vi "HeaderAction.vi"(0 "InstrClass":refnum<class "CoboltMLD.lvclass"> caption="DNL_LabVIEW Object in", 11 "error in (no error)":errorcluster caption="entrée d'erreur (pas d'erreur)") -> (4 "InstrClassOut":refnum<class "CoboltMLD.lvclass"> caption="DNL_LabVIEW Object out", 6 "DataNames":string[](array[string]), 8 "Instr Name":string, 10 "HeaderString":string, 13 "ArrDisplayNames":string[](array[string]), 14 "DisplayNames":string[](array[string]), 15 "error out":errorcluster caption="sortie d'erreur")   [LabVIEW 2019, in "CoboltMLD.lvclass"]
uses:
  CoboltMLD.lvclass
  C:/Programmes Labview/LabScanV1A/DevicesClass/BaseDevice/BaseDevice.lvclass
  <userlib>/TaikoLaser/PDLM_LaserMode.ctl
  CoboltMLD.lvclass/CoboltMLD.ctl
  <userlib>/GenProg/ReadValByRefDbl.vi
  <userlib>/GenProg/ReadValByRefBool.vi
  <userlib>/GenProg/ReadValByRefU32.vi
  <userlib>/GenProg/ReadValByRefString.vi
  <vilib>/Utility/error.llb/Error Cluster From Error Code.vi
  <vilib>/ErrorRing/Error Ring.xnode
  BaseDevice/BaseDevice.lvclass
panel:
  in  "LaserMode":T1
  out "InfoStr":string
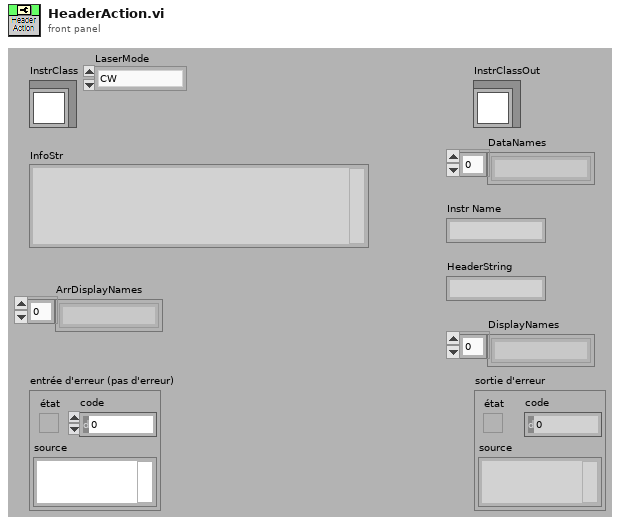
[diagram p1: front panel]
types:
  T1 = typedef "PDLM_LaserMode.ctl" = enum32{"CW", "PULSE", "BURST"}
  T2 = typedef "CoboltMLD.lvclass/CoboltMLD_Func.ctl" = enum16{"Power (mW)", "Current (mA)"}
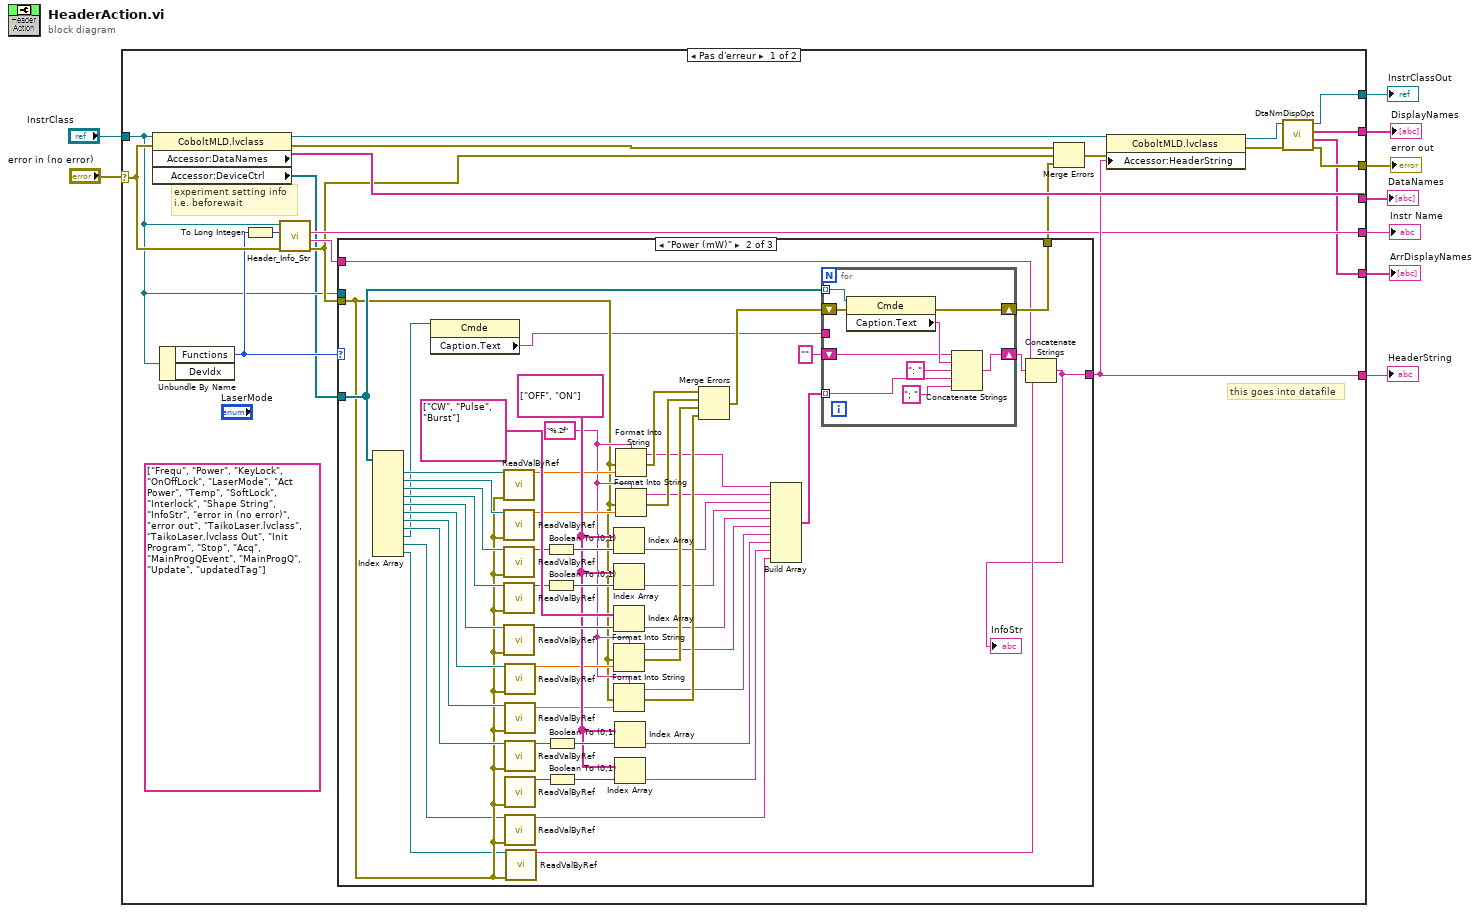
[diagram p0: block diagram]
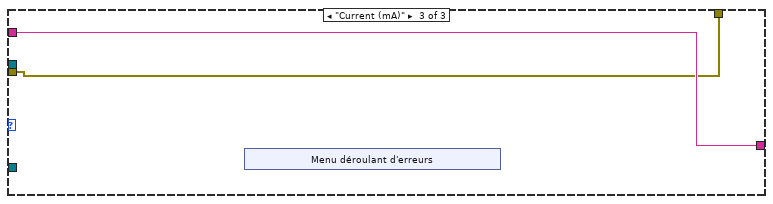
[diagram p3: hidden frame]
diagram:
  n1 = case shown="Pas d'erreur" "error in (no error)" {
    selector: "error in (no error)" -> [w18 w100]
    tunnel: [w26 _] -> w8
    tunnel: [w29 _] -> w7
    tunnel: "InstrClass" -> [w11 w101]
    tunnel: [w24 w100] -> w5
    tunnel: [w23 w101] -> w3
    tunnel: [w20 _] -> w4
    tunnel: [w21 _] -> w2
    tunnel: [w14 _] -> w1
    frame No Error {
      (unwired) string[] ["Frequ", "Power", "KeyLock", "OnOffLock", "LaserMode", "Act Power", "Temp", "SoftLock", "Interlock", "Shape String", "InfoStr", "error in (no error)", "error out", "TaikoLaser.lvclass", "TaikoLaser.lvclass Out", "Init Program", "Stop", "Acq", "MainProgQEvent", "MainProgQ", "Update", "updatedTag"] ("ControlsNames")
      # "this goes into datafile"
      # "experiment setting info\ni.e. beforewait"
      n2 = property class="CoboltMLD.lvclass"(reference=w11, error in=w18) -> (reference out=w28:refnum<class "CoboltMLD.lvclass">, error out=w27:errorcluster, "Accessor:DataNames"=w29:string[], "Accessor:DeviceCtrl"=w10:refnum<vi>[])
      n3 = Unbundle By Name(w11) -> ("Functions"=w16:T2)  [unwired: 1 out]
      n4 = To Long Integer(number=w16) -> (32bit integer=w15:i32)
      n5 = call-dynamic "Header_Info_Str.vi"("error in (no error)"=w18, "Functions"=w15, "DefaultDev in"=w11) -> ("error out"=w13:errorcluster, "HdrInfoStr"=w19:string, "InstrumentName"=w20:string)  [unwired: 5 in, 1 out]
      n6 = case shown="\"Power (mW)\"" w16 {
        tunnel: [w31 w38 w94] -> w26
        tunnel: w19 -> [w31 w33 w94]
        tunnel: w13 -> [w30 w42 w93]
        tunnel: [w30 w39 w93] -> w12
        tunnel: w11 -> [_ _ _]
        tunnel: w10 -> [_ w83 _]
        frame Default {
        }
        frame "Power (mW)" {
          w60 = "%.2f" ("chaîne de format")
          w66 = string[] ["OFF", "ON"] ("ControlsNames")
          n7 = Index Array(array=w83) -> (element #1=w82:refnum<vi>, element #2=w81:refnum<vi>, element #3=w80:refnum<vi>, element #4=w79:refnum<vi>, element #5=w78:refnum<vi>, element #6=w75:refnum<vi>, element #7=w65:refnum<vi>, element #8=w64:refnum<vi>, element #9=w35:refnum<vi>, element #10=w37:refnum<vi>, element #11=w36:refnum<vi>)  [unwired: 11 in]
          n8 = property class="Cmde"(reference=w35) -> ("Caption.Text"=w34:string)  [unwired: 1 in, 2 out]
          n9 = call-poly <userlib>:"ReadValByRef.vi"("Control Ref"=w82, "error in"=w42) -> ("Valeur"=w63:dbl)  [unwired: 12 in, 1 out]
          n10 = call-poly <userlib>:"ReadValByRef.vi"("Control Ref"=w81, "error in"=w42) -> ("Valeur"=w62:dbl)  [unwired: 12 in, 1 out]
          n11 = call-poly <userlib>:"ReadValByRef.vi"("Control Ref"=w80, "error in"=w42) -> ("Valeur"=w74:bool)  [unwired: 12 in, 1 out]
          n12 = call-poly <userlib>:"ReadValByRef.vi"("Control Ref"=w79, "error in"=w42) -> ("Valeur"=w73:bool)  [unwired: 12 in, 1 out]
          n13 = call-poly <userlib>:"ReadValByRef.vi"("Control Ref"=w78, "error in"=w42) -> ("Valeur"=w77:u32)  [unwired: 12 in, 1 out]
          n14 = call-poly <userlib>:"ReadValByRef.vi"("Control Ref"=w75, "error in"=w42) -> ("Valeur"=w61:dbl)  [unwired: 12 in, 1 out]
          n15 = call-poly <userlib>:"ReadValByRef.vi"("Control Ref"=w65, "error in"=w42) -> ("Valeur"=w59:dbl)  [unwired: 12 in, 1 out]
          n16 = call-poly <userlib>:"ReadValByRef.vi"("Control Ref"=w64, "error in"=w42) -> ("Valeur"=w70:bool)  [unwired: 12 in, 1 out]
          n17 = call-poly <userlib>:"ReadValByRef.vi"("error in"=w42) -> ("Valeur"=w69:bool)  [unwired: 13 in, 1 out]
          n18 = call-poly <userlib>:"ReadValByRef.vi"("Control Ref"=w37, "error in"=w42) -> ("Valeur"=w45:string)  [unwired: 12 in, 1 out]
          n19 = call-poly <userlib>:"ReadValByRef.vi"("Control Ref"=w36, "error in"=w42) -> ("Valeur"=w40:string)  [unwired: 12 in, 1 out]
          n20 = Boolean To (0,1)(Boolean=w74) -> (0, 1=w71:i16)
          n21 = Boolean To (0,1)(Boolean=w73) -> (0, 1=w72:i16)
          n22 = Boolean To (0,1)(Boolean=w70) -> (0, 1=w67:i16)
          n23 = Boolean To (0,1)(Boolean=w69) -> (0, 1=w68:i16)
          n24 = Index Array(array=w66, index=w71) -> (element=w52:string)
          n25 = Index Array(array=w66, index=w72) -> (element=w51:string)
          n26 = Index Array(array=string[] ["CW", "Pulse", "Burst"] ("ControlsNames"), index=w77) -> (element=w50:string)
          n27 = Format Into String(format string=w60, error in=w42, w61) -> (resulting string=w49:string, error out=w56:errorcluster)  [unwired: 1 in]
          n28 = Format Into String(format string=w60, error in=w42, w59) -> (resulting string=w48:string, error out=w55:errorcluster)  [unwired: 1 in]
          n29 = Index Array(array=w66, index=w67) -> (element=w47:string)
          n30 = Index Array(array=w66, index=w68) -> (element=w46:string)
          n31 = Format Into String(format string=w60, error in=w42, w63) -> (resulting string=w54:string, error out=w58:errorcluster)  [unwired: 1 in]
          n32 = Format Into String(format string=w60, error in=w42, w62) -> (resulting string=w53:string, error out=w57:errorcluster)  [unwired: 1 in]
          n33 = Merge Errors(w58, w57, w56, w55) -> (w43:errorcluster)
          n34 = Build Array(w54, w53, w52, w51, w50, w49, w48, w47, w46, w45) -> (w44:string[])
          n35 = for {
            tunnel: w83 -> [w92] mode=indexing
            shift-right: [w90] -> w39
            shift-left: w43 -> [w91]
            tunnel: w44 -> [w87] mode=indexing
            shift-right: [w85] -> w41
            shift-left: "" -> [w84]
            tunnel: w34 -> [_]
            n36 = property class="Cmde"(reference=w92, error in=w91) -> (error out=w90:errorcluster, "Caption.Text"=w89:string)  [unwired: 1 out]
            n37 = Concatenate Strings(w84, w89, ": " ("chaîne"), w87, "; " ("chaîne")) -> (w85:string)
          }
          n38 = Concatenate Strings(w33, w41, w40) -> (w38:string)
          "InfoStr" <- w38
        }
        frame "Current (mA)" {
          n39 = xnode "Menu déroulant d'erreurs"() -> ()  [unwired: 1 out]
        }
      }
      n40 = Merge Errors(w27, w13, w12) -> (w17:errorcluster)
      n41 = property class="CoboltMLD.lvclass"(reference=w28, error in=w17, "Accessor:HeaderString"=w26) -> (reference out=w22:refnum<class "CoboltMLD.lvclass">, error out=w25:errorcluster)
      n42 = call "DtaNmDispOpt.vi"("error in (no error)"=w25, "BaseDevice en entrée"=w22) -> ("error out"=w24:errorcluster, "ArrDisplayNames"=w14:string[], "DisplayNames"=w21:string[], "BaseDevice en sortie"=w23:refnum<class "CoboltMLD.lvclass">)  [unwired: 6 in]
    }
    frame Error {
    }
  }
  "error out" <- w5
  "InstrClassOut" <- w3
  "DataNames" <- w7
  "HeaderString" <- w8
  "Instr Name" <- w4
  "DisplayNames" <- w2
  "ArrDisplayNames" <- w1
